vi "Port.vi"(11 "URI in":refnum<class "URI.lvclass">) -> (2 "Port":u16, 3 "URI out":refnum<class "URI.lvclass">, 5 "Unset":bool)   [LabVIEW 2020, in "URI.lvlib" / "URI.lvclass"]
uses:
  URI.lvclass
  URI.lvclass/URI.ctl
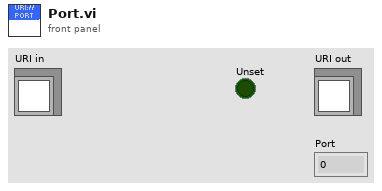
[diagram p1: front panel]
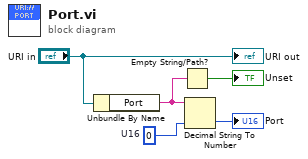
[diagram p0: block diagram]
diagram:
  w3 = u16 0  # U16
  n1 = Unbundle By Name("URI in") -> ("Port"=w4:string)
  n2 = Empty String/Path?(string/path=w4) -> (empty?=→"Unset":bool)
  n3 = Decimal String To Number(string=w4, default (0L)=w3) -> (number=→"Port":u16)  [unwired: 1 in, 1 out]
  "URI out" <- "URI in"
